vi "Validate Fixed Header.vi"(8 "error in (no error)":errorcluster, 11 "ControlPacket in":refnum<class "ControlPacket.lvclass">) -> (0 "error out":errorcluster, 1 "Valid":bool, 3 "ControlPacket out":refnum<class "ControlPacket.lvclass">)   [LabVIEW 2013, in "MQTT_Control_Packets.lvlib" / "ControlPacket.lvclass"]
uses:
  ControlPacket.lvclass
  ControlPacket.lvclass/ControlPacket.ctl
  MQTT_311/MQTTVersion.lvclass
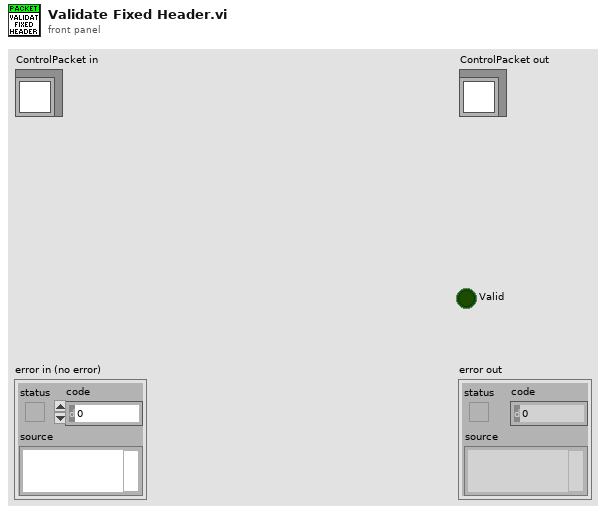
[diagram p1: front panel]
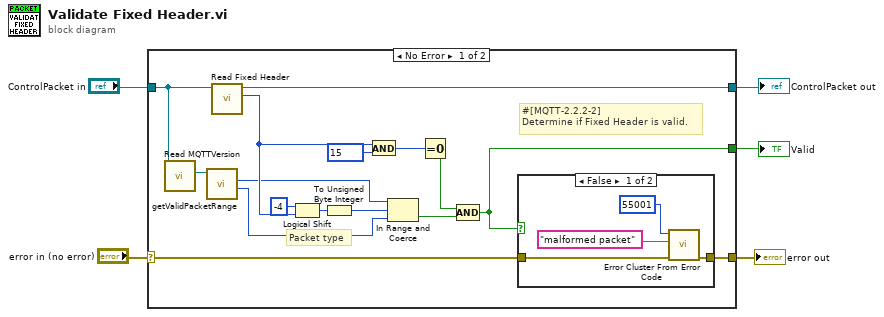
[diagram p0: block diagram]
diagram:
  n1 = case shown="No Error" "error in (no error)" {
    selector: "error in (no error)" -> [w19 w28]
    tunnel: [w18 w28] -> w4
    tunnel: [w10 _] -> w1
    tunnel: [w21 w27] -> w2
    tunnel: "ControlPacket in" -> [w9 w27]
    frame No Error {
      # "#[MQTT-2.2.2-2]\nDetermine if Fixed Header is valid."
      # "Packet type"
      n2 = call "Read MQTTVersion.vi"("ControlPacket in"=w9) -> ("MQTTVersion"=w8:refnum<class "MQTTVersion.lvclass">)  [unwired: 9 in, 1 out]
      n3 = call-dynamic "getValidPacketRange.vi"("MQTTVersion in"=w8) -> ("Lower Range"=w6:u8, "Upper Range"=w7:u8)  [unwired: 8 in, 1 out]
      n4 = call "Read Fixed Header.vi"("ControlPacket in"=w9) -> ("Fixed Header"=w13:u8, "ControlPacket out"=w21:refnum<class "ControlPacket.lvclass">)  [unwired: 9 in]
      n5 = Logical Shift(y=i16 -4, x=w13) -> (x << y=w15:u8)
      n6 = To Unsigned Byte Integer(number=w15) -> (unsigned 8bit integer=w14:u8)
      n7 = And(x=w13, y=u8 15) -> (x .and. y?=w17:u8)
      n8 = In Range and Coerce(upper limit=w7, x=w14, lower limit=w6) -> (In Range?=w12:bool)  [unwired: 1 out]
      n9 = Equal To 0?(x=w17) -> (x = 0?=w11:bool)
      n10 = Compound Arithmetic op=AND(w11, w12) -> (w10:bool)
      n11 = case shown="False" w10 {
        tunnel: [w23 w26] -> w18
        tunnel: w19 -> [w22 w26]
        frame False {
          n12 = call <vilib>:"Error Cluster From Error Code.vi"("error in (no error)"=w22, "error message (\"\")"="malformed packet" ("error message (\"\")"), "error code (0)"=55001) -> ("error out"=w23:errorcluster)  [unwired: 6 in]
        }
        frame True {
        }
      }
    }
    frame Error {
    }
  }
  "Valid" <- w1
  "error out" <- w4
  "ControlPacket out" <- w2
